vi "Lidar Code with XY graph.vi"() -> ()   [LabVIEW 2016]
uses:
  <instrlib>/Hokuyo URG Series/Public/Initialize-cRIO-USB.vi
  <instrlib>/Hokuyo URG Series/Hokuyo URG Series.lvlib
panel:
  in  "Boolean":bool
  out "Array 2":dbl[](array[numeric])
  in  "Array":dbl[](array[numeric])
  out "XY Graph":cluster{"Y":dbl[], "Y":dbl[]}[](graph)
  in  "polar attributes (hidden)":T1={"maximum"=30000.0, "minimum"=0.0, "clip to min"=FALSE, "log?(F)"=TRUE, "grid color"=6710886, "plot color"=65280, "fmt and prec"={"format"=enum."Decimal", "precision"=0}, "visible section"=8} {"minimum" format="%0.2f"; "maximum" format="%0.2f"}
  in  "Protocol":u32(ring)=2 items=["Convert to Latest", "SCIP 1.1", "SCIP 2.0"]
  in  "ID Query?":bool=TRUE
  in  "Checksum":bool
  in  "Stop":bool
  out "Data Aquired":picture
  in  "Grid Color":u32(colorbox)=16777222
  in  "Plot Color":u32(colorbox)=6618880
  in  "Max (m)":dbl=4.1
  in  "End Point":dbl=120.0
  in  "Start Point":dbl=-120.0
  in  "Cluster Count":dbl=1.0
  in  "Encoding Width":u16(ring)=3 items=["2 Byte"=2, "3 Byte"=3]
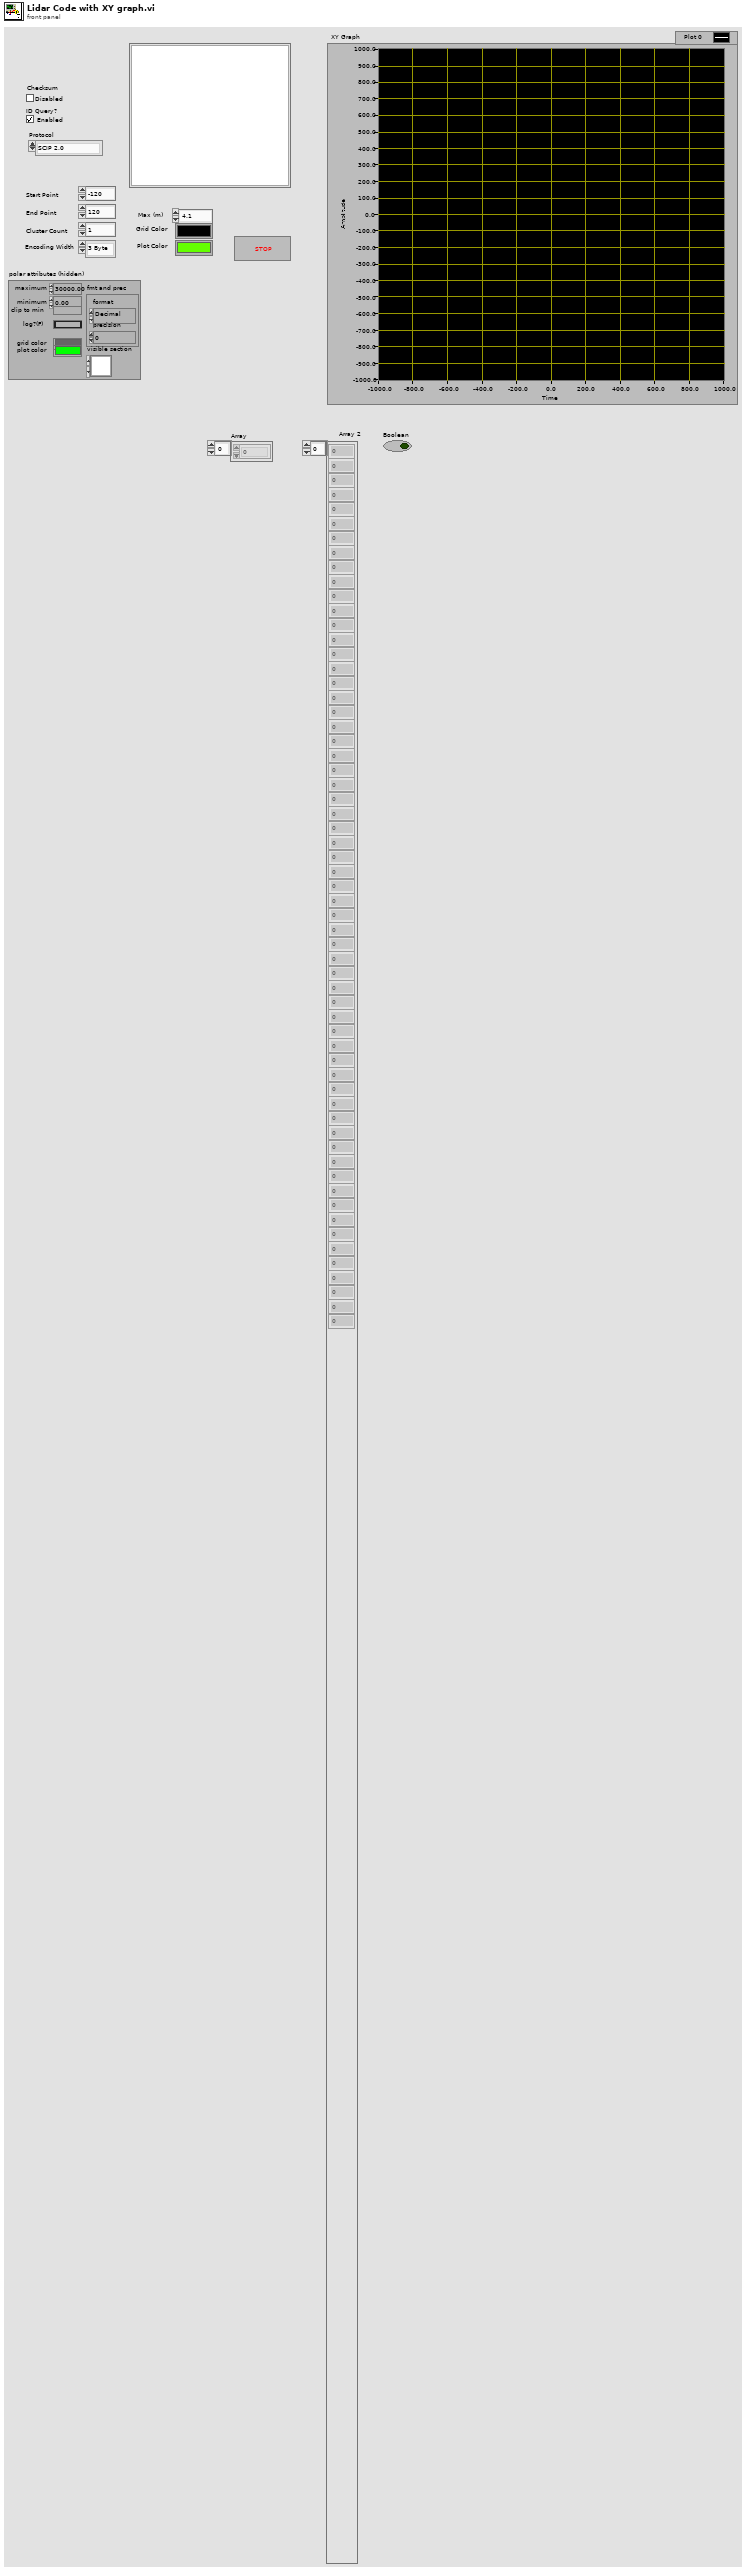
[diagram p1: front panel]
types:
  T1 = cluster{"maximum":dbl, "minimum":dbl, "clip to min":bool, "log?(F)":bool, "grid color":u32, "plot color":u32, "fmt and prec":cluster{"format":enum8{"Decimal", "Scientific", "Engineering", "Binary", "Octal", "Hex"}, "precision":u8}, "visible section":u16}
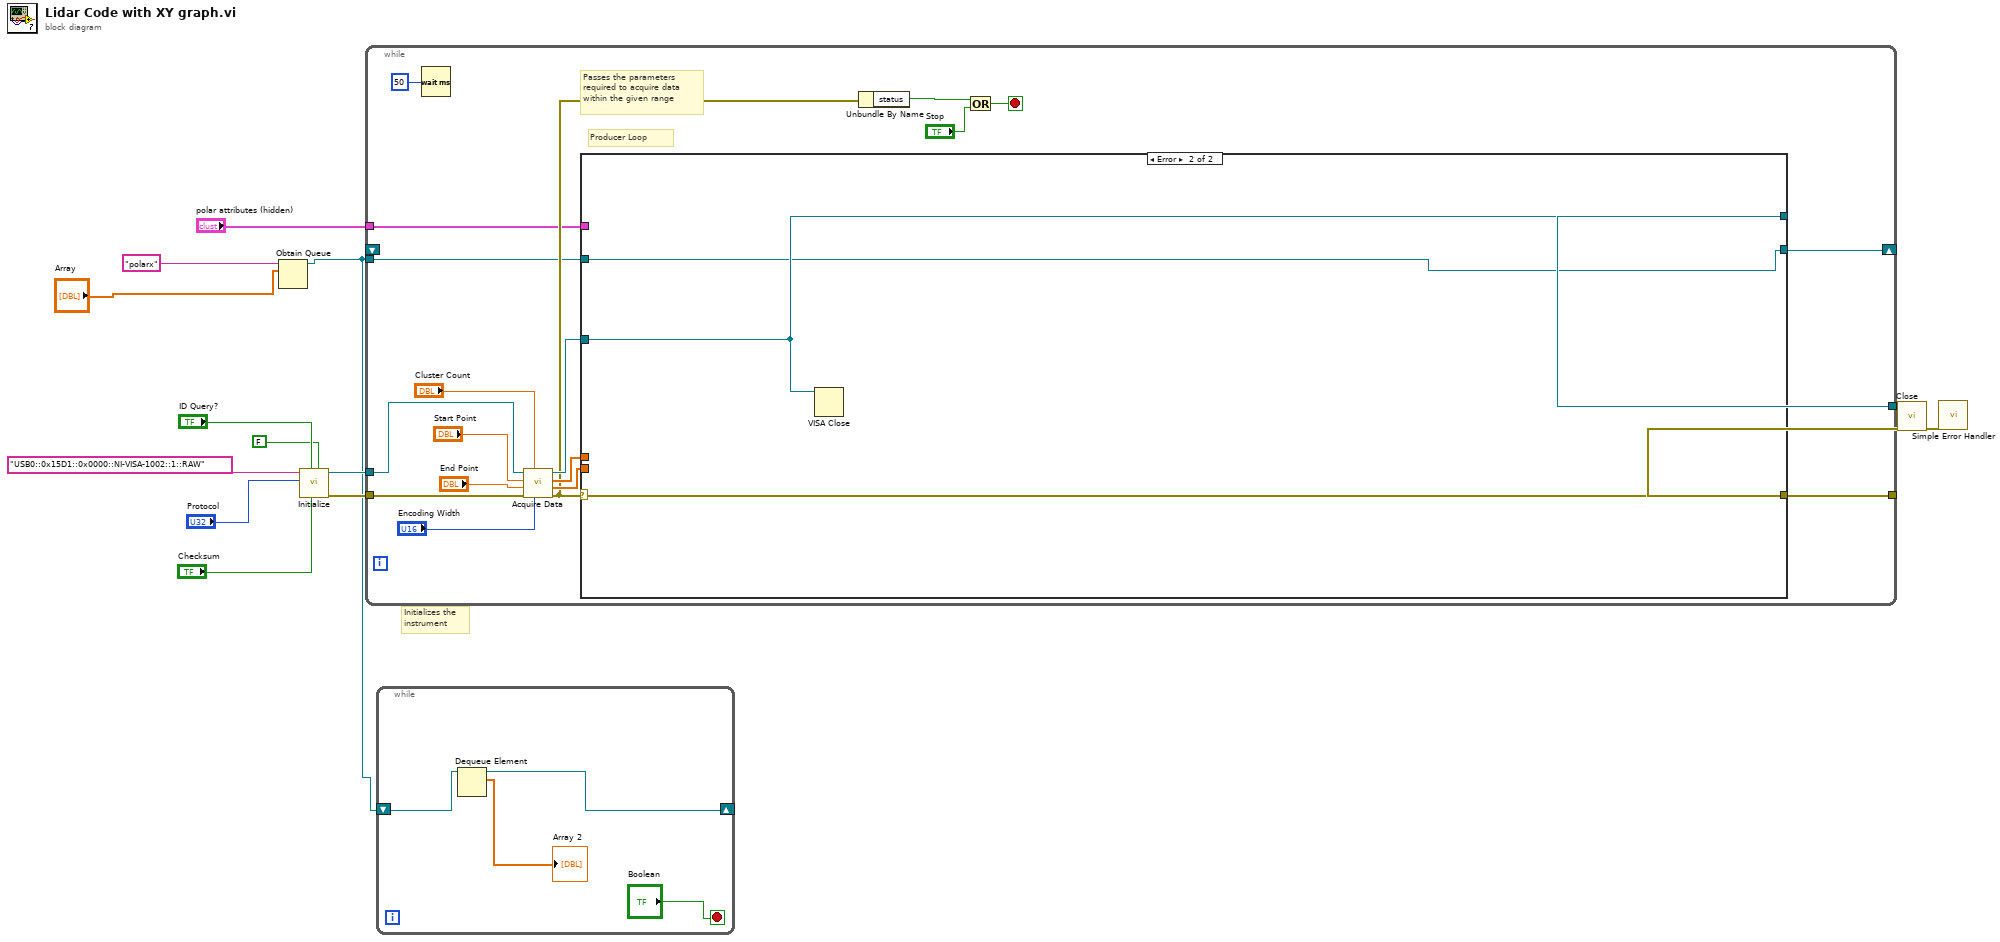
[diagram p0: block diagram]
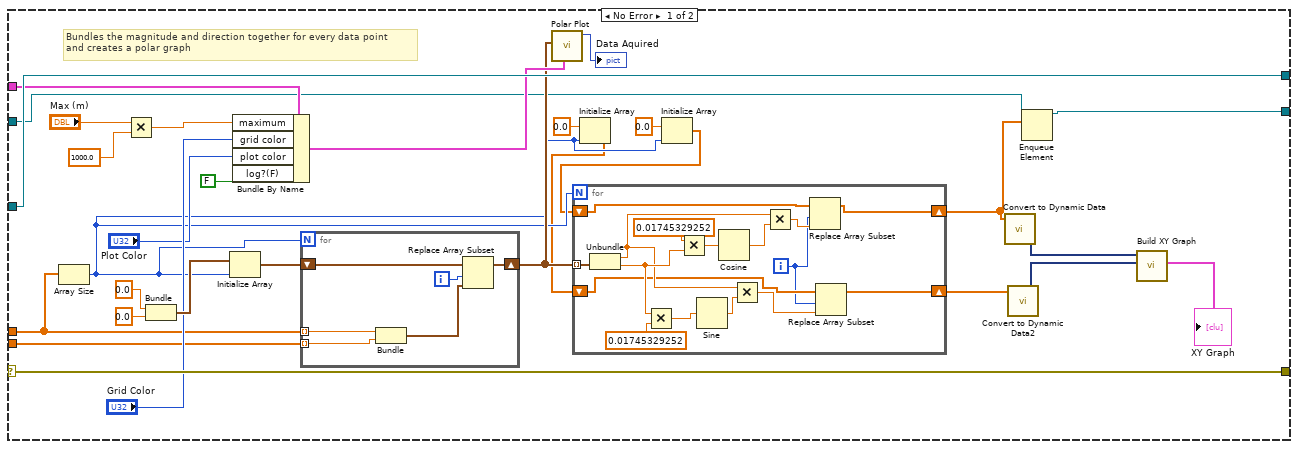
[diagram p2: hidden frame]
diagram:
  # "Initializes the instrument"
  n1 = Obtain Queue(name (unnamed)="polarx", element data type="Array") -> (queue out=w1:refnum<queue>)  [unwired: 3 in, 2 out]
  n2 = call-poly <instrlib>:"Initialize.vi"("Reset? (F: No)"=FALSE ("Reset Instrument (Disabled)"), "Checksum (Disabled)"="Checksum", "ID Query? (Enabled)"="ID Query?", "Protocol (2: SCIP 2.0)"="Protocol", "VISA resource name"="USB0::0x15D1::0x0000::NI-VISA-1002::1::RAW") -> ("error out"=w7:errorcluster, "VISA resource name out"=w8:refnum<visa-resource-name>)  [unwired: 5 in]
  n3 = while {
    tunnel: w8 -> [w23]
    tunnel: [w18] -> w14
    tunnel: w7 -> [w22]
    tunnel: "polar attributes (hidden)" -> [w21]
    tunnel: [w17] -> w4
    tunnel: w1 -> [w16]
    shift-right: [w15] -> _
    shift-left: _ -> [_]
    stop <- w31 stop-if-true
    # "Producer Loop"
    # "Passes the parameters\nrequired to acquire data\nwithin the given range"
    n4 = Wait (ms)(milliseconds to wait=u32 50) -> ()  [unwired: 1 out]
    n5 = call <instrlib>:"Acquire Data.vi"("Data Encoding Width (3 Byte)"="Encoding Width", "Cluster Count (1)"="Cluster Count", "error in (no error)"=w22, "End Point (120°)"="End Point", "Start Point (-120°)"="Start Point", "VISA resource name"=w23) -> ("error out"=w27:errorcluster, "Direction"=w28:dbl[], "Magnitude"=w29:dbl[], "VISA resource name out"=w30:refnum<visa-resource-name>)  [unwired: 2 in]
    n6 = case shown="Error" w27 {
      selector: w27 -> [w61 w88]
      tunnel: [w61 w88] -> w18
      tunnel: w30 -> [w62 w87]
      tunnel: [w62 w87] -> w17
      tunnel: w29 -> [w47 _]
      tunnel: w28 -> [w48 _]
      tunnel: w21 -> [w55 _]
      tunnel: w16 -> [w35 w86]
      tunnel: [w36 w86] -> w15
      frame No Error {
        # "Bundles the magnitude and direction together for every data point\nand creates a polar graph"
        n7 = Array Size(array=w47) -> (size(s)=w43:i32)
        n8 = Multiply(x="Max (m)", y=1000.0) -> (x*y=w51:dbl)
        n9 = Bundle(0.0, 0.0) -> (w58:cluster{dbl, dbl})  [unwired: 1 in]
        n10 = Initialize Array(w58, w43) -> (w57:cluster{dbl, dbl}[])
        n11 = Bundle By Name(cluster=w55, "maximum"=w51, "grid color"="Grid Color", "plot color"="Plot Color", "log?(F)"=FALSE) -> (w56:T1)
        n12 = for {
          N: w43 -> [_]
          shift-right: [w81] -> w46
          shift-left: w57 -> [w82]
          tunnel: w47 -> [w85] mode=indexing
          tunnel: w48 -> [w84] mode=indexing
          i -> [w83]
          n13 = Bundle(w85, w84) -> (w80:cluster{dbl, dbl})  [unwired: 1 in]
          n14 = Replace Array Subset(array=w82, new element=w80, index=w83) -> (w81:cluster{dbl, dbl}[])
        }
        n15 = call <vilib>:"Polar Plot.vi"("polar attributes"=w56, "data array [mag, phase (deg)]"=w46) -> ("new picture"=→"Data Aquired":picture)  [unwired: 9 in]
        n16 = Initialize Array(0.0 ("element"), w43) -> (w41:dbl[])
        n17 = Initialize Array(0.0 ("element"), w43) -> (w42:dbl[])
        n18 = for {
          N: w43 -> [_]
          tunnel: w46 -> [w79] mode=indexing
          shift-right: [w65] -> w34
          shift-left: w42 -> [w74]
          shift-right: [w64] -> w38
          shift-left: w41 -> [w67]
          i -> [w66]
          n19 = Unbundle(w79) -> (w69:dbl, w70:dbl)
          n20 = Multiply(x=w70, y=0.01745329252 ("x")) -> (x*y=w72:dbl)
          n21 = Multiply(x=0.01745329252, y=w70) -> (x*y=w76:dbl)
          n22 = Sine(x=w72) -> (sin(x)=w73:dbl)
          n23 = Cosine(x=w76) -> (cos(x)=w77:dbl)
          n24 = Multiply(x=w69, y=w73) -> (x*y=w68:dbl)
          n25 = Multiply(x=w69, y=w77) -> (x*y=w78:dbl)
          n26 = Replace Array Subset(array=w74, new element=w78, index=w66) -> (w65:dbl[])
          n27 = Replace Array Subset(array=w67, new element=w68, index=w66) -> (w64:dbl[])
        }
        n28 = call "Convert to Dynamic Data"("Array"=w34) -> ("Dynamic Data Type"=w39:dynamicdata)  [unwired: 3 in]
        n29 = call "Convert to Dynamic Data2"("Array"=w38) -> ("Dynamic Data Type"=w37:dynamicdata)  [unwired: 3 in]
        n30 = Enqueue Element(queue=w35, element=w34) -> (queue out=w36:refnum<queue>)  [unwired: 2 in, 2 out]
        n31 = call "Build XY Graph"("Y Input"=w37, "X Input"=w39) -> ("XY Graph"=→"XY Graph":cluster{"X":dbl[], "Y":dbl[]}[])  [unwired: 8 in, 1 out]
      }
      frame Error {
        n32 = VISA Close(VISA resource name=w87) -> ()  [unwired: 1 in, 1 out]
      }
    }
    n33 = Unbundle By Name(w27) -> ("status"=w33:bool)
    n34 = Or(x=w33, y="Stop") -> (x .or. y?=w31:bool)
  }
  n35 = while {
    shift-right: [w90] -> _
    shift-left: w1 -> [w91]
    stop <- "Boolean" stop-if-true
    n36 = Dequeue Element(queue=w91) -> (queue out=w90:refnum<queue>, element=→"Array 2":dbl[])  [unwired: 2 in, 2 out]
  }
  n37 = call <instrlib>:"Close.vi"("error in (no error)"=w14, "VISA resource name"=w4) -> ("error out"=w12:errorcluster)  [unwired: 9 in]
  n38 = call <vilib>:"Simple Error Handler.vi"("error in (no error)"=w12) -> ()  [unwired: 4 in, 5 out]
